vi "generate system name.vi"(10 "queue":T1, 11 "network hostname":string="localhost") -> (3 "queue name":string)   [LabVIEW 2013, in "module execution process.lvlib"]
uses:
  module execution process.lvlib
  queue name.ctl
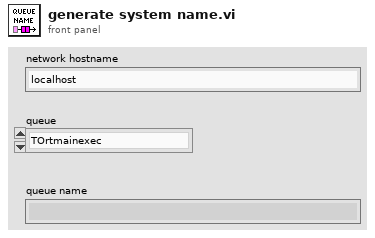
[diagram p1: front panel]
types:
  T1 = typedef "module execution process.lvlib/queue name.ctl" = enum16{"TOrtmainexec", "FROMrtmainexec"}
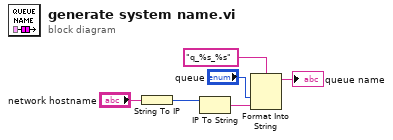
[diagram p0: block diagram]
diagram:
  n1 = String To IP(1:"network hostname") -> (0:w4:u32)
  n2 = IP To String(2:w4) -> (0:w2:string)  [unwired: 1 in]
  n3 = Format Into String(format string="q_%s_%s", "queue", w2) -> (resulting string=→"queue name":string)  [unwired: 2 in, 1 out]
